vi "stop.vi"(8 "error in (no error)":errorcluster, 11 "Hamamatsu_C9100-13 in":refnum<class "Hamamatsu_C9100-13.lvclass">) -> (0 "error out":errorcluster, 3 "Hamamatsu_C9100-13 out":refnum<class "Hamamatsu_C9100-13.lvclass">)   [LabVIEW 2013, in "Hamamatsu_C9100-13.lvclass"]
uses:
  Hamamatsu_C9100-13.lvclass
  Hamamatsu_C9100-13.lvclass/Hamamatsu_C9100-13.ctl
  Camera.lvclass
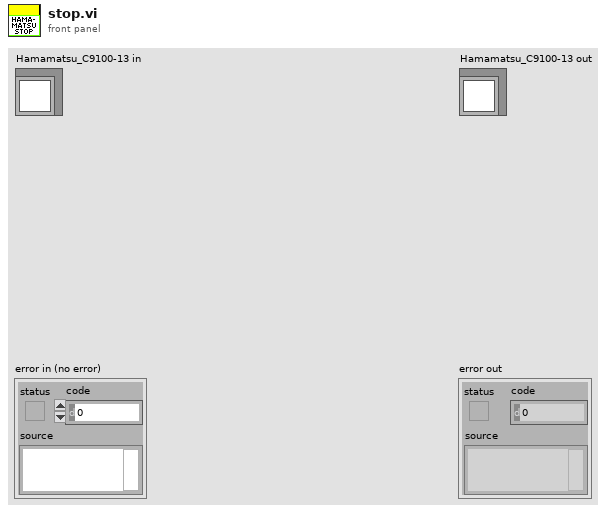
[diagram p1: front panel]
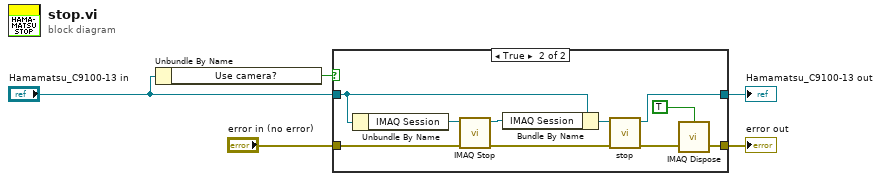
[diagram p0: block diagram]
diagram:
  n1 = Unbundle By Name("Hamamatsu_C9100-13 in") -> ("Use camera?"=w1:bool)
  n2 = case shown="True" w1 {
    tunnel: [w7 w17] -> w5
    tunnel: "error in (no error)" -> [w6 w16]
    tunnel: [w6 w8] -> w3
    tunnel: "Hamamatsu_C9100-13 in" -> [w7 w14]
    frame False {
    }
    frame True {
      n3 = Unbundle By Name(w14) -> ("IMAQ Session"=w15:refnum<k11>)
      n4 = call <vilib>:"IMAQ Stop.vi"("error in (no error)"=w16, "IMAQ Session In"=w15) -> ("error out"=w10:errorcluster, "IMAQ Session Out"=w12:refnum<k11>)  [unwired: 8 in]
      n5 = Bundle By Name(cluster=w14, "IMAQ Session"=w12) -> (w13:refnum<class "Hamamatsu_C9100-13.lvclass">)
      n6 = call-parent "stop.vi"("error in (no error)"=w10, "Camera in"=w13) -> ("error out"=w9:errorcluster, "Camera out"=w17:refnum<class "Hamamatsu_C9100-13.lvclass">)  [unwired: 8 in]
      n7 = call "IMAQ Dispose"("All Images? (No)"=TRUE, "error in (no error)"=w9) -> ("error out"=w8:errorcluster)  [unwired: 4 in]
    }
  }
  "error out" <- w3
  "Hamamatsu_C9100-13 out" <- w5
